vi "SW_Get_1D_Array_mean.vi"(1 "1D array":dbl[](array[numeric])) -> (0 "Mean of 1D Array":dbl)   [LabVIEW 2018, in "Tracker.lvlib"]
uses:
  Tracker.lvlib
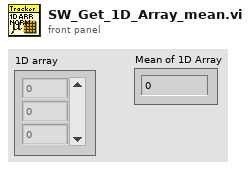
[diagram p1: front panel]
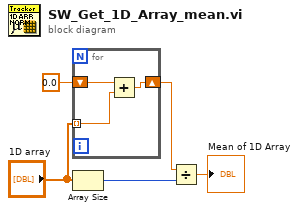
[diagram p0: block diagram]
diagram:
  n1 = for {
    tunnel: "1D array" -> [w8] mode=indexing
    shift-right: [w7] -> w4
    shift-left: 0.0 -> [w6]
    n2 = Add(x=w6, y=w8) -> (x+y=w7:dbl)
  }
  n3 = Array Size(array="1D array") -> (size(s)=w2:i32)
  n4 = Divide(x=w4, y=w2) -> (x/y=→"Mean of 1D Array":dbl)
